vi "Port to index p.vi"   [LabVIEW 2010]
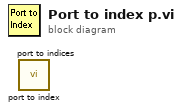
[diagram p0: block diagram]
diagram:
  n1 = call "port to index.vi"() -> ()  [unwired: 11 in, 1 out]
  n2 = call "port to indices.vi"() -> ()  [unwired: 11 in, 1 out]
